vi "Append_array.vi"(8 "elem2":dbl, 9 "Array2":dbl[](array[numeric]), 10 "elem1":dbl, 11 "array1":dbl[](array[numeric])) -> (1 "output array2":dbl[](array[numeric]), 3 "output array1":dbl[](array[numeric]))   [LabVIEW 2017]
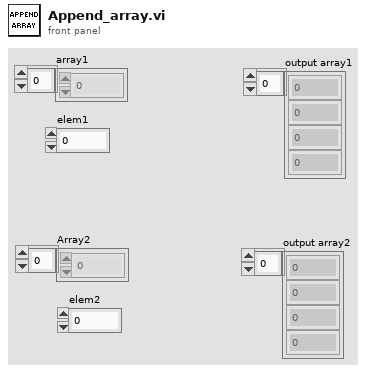
[diagram p1: front panel]
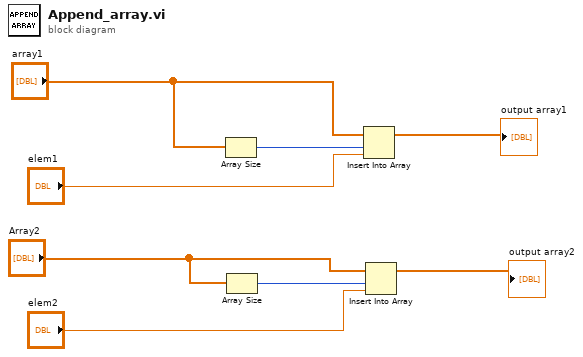
[diagram p0: block diagram]
diagram:
  n1 = Array Size(array="array1") -> (size(s)=w2:i32)
  n2 = Array Size(array="Array2") -> (size(s)=w1:i32)
  n3 = Insert Into Array(array="array1", index=w2, new element="elem1") -> (→"output array1":dbl[])
  n4 = Insert Into Array(array="Array2", index=w1, new element="elem2") -> (→"output array2":dbl[])
